vi "PH_SHS_Analysis.evt call Set SHS Device Config.vi"(0 "i ref in":refnum<vi>, 1 "Instance":string, 2 "SHS Device Config":T1={"focal length [m]"=0.010000000000000009, "pixel size [m/px]"=6.7e-06, "wavelength [m]"=1.053e-06} {"wavelength [m]" format="%#_6p"; "pixel size [m/px]" format="%#_6p"; "focal length [m]" format="%#_6p"}, 5 "error in (no error)":errorcluster) -> (14 "i ref out":refnum<vi>, 19 "error out":errorcluster)   [LabVIEW 2014, in "PH_SHS_Analysis.lvlib"]
doc: "This VI calls the event case \"SetSHSDevConfig\" by a simple call."
uses:
  PH_SHS_Analysis.lvlib
  User/Eisenbarth/SHS_v4/SHS_Analysis/SHS_DeviceConfig.ctl
  CSCore/CSSystem/CoreLib/CoreLib.double 2 byte array.vi
  CSCore/CSSystem/CoreLib/CoreLib.lvlib
  CSCore/BaseProcess/BaseProcess.lvlib
  User/Eisenbarth/SHS_v4/SHS_Analysis/SHS_Analysis.lvlib
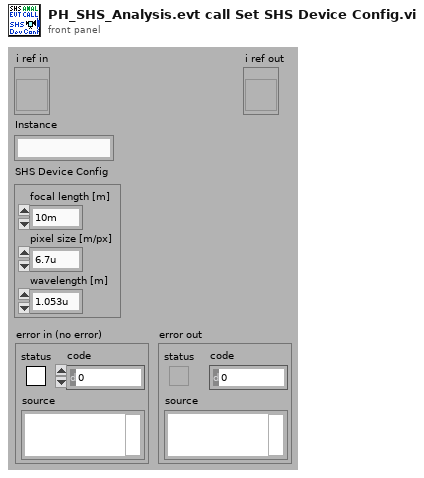
[diagram p1: front panel]
types:
  T1 = typedef "SHS_Analysis.lvlib/SHS_DeviceConfig.ctl" = cluster{"focal length [m]":dbl, "pixel size [m/px]":dbl, "wavelength [m]":dbl}
  T2 = typedef "CoreDefs.rawDataType.ctl" = i8[]
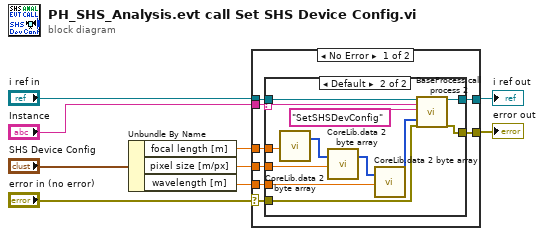
[diagram p0: block diagram]
diagram:
  n1 = Unbundle By Name("SHS Device Config") -> ("focal length [m]"=w3:dbl, "pixel size [m/px]"=w2:dbl, "wavelength [m]"=w1:dbl)
  n2 = case shown="No Error" "error in (no error)" {
    selector: "error in (no error)" -> [w14 w32]
    tunnel: [w17 w33] -> w6
    tunnel: [w16 w32] -> w5
    tunnel: "i ref in" -> [w15 w33]
    tunnel: "Instance" -> [w13 _]
    tunnel: w3 -> [w12 _]
    tunnel: w2 -> [w11 _]
    tunnel: w1 -> [w10 _]
    frame No Error {
      n3 = case shown="Default" w13 {
        selector: w13 -> [_ w25]
        tunnel: [w19 w30] -> w17
        tunnel: [w18 w29] -> w16
        tunnel: w15 -> [w19 w28]
        tunnel: w14 -> [w18 w26]
        tunnel: w12 -> [_ w24]
        tunnel: w11 -> [_ w22]
        tunnel: w10 -> [_ w21]
        frame "N/A" {
        }
        frame Default {
          n4 = call-poly "CoreLib.data 2 byte array.vi"("f64"=w24) -> ("byteArray out"=w23:T2)  [unwired: 18 in]
          n5 = call-poly "CoreLib.data 2 byte array.vi"("byteArray"=w23, "f64"=w22) -> ("byteArray out"=w20:T2)  [unwired: 17 in]
          n6 = call-poly "CoreLib.data 2 byte array.vi"("byteArray"=w20, "f64"=w21) -> ("byteArray out"=w27:T2)  [unwired: 17 in]
          n7 = call "BaseProcess.call process 2.vi"("i ref in"=w28, "Object"=w25, "Selector"="SetSHSDevConfig", "Data"=w27, "error in (no error)"=w26) -> ("i ref out"=w30:refnum<vi>, "error out"=w29:errorcluster)  [unwired: 13 in]
        }
      }
    }
    frame Error {
    }
  }
  "i ref out" <- w6
  "error out" <- w5
